vi "Partition_Sort.vi"(8 "FreezeIdx":i32[](array[numeric]), 9 "PartitionArray":string[](array[string]), 10 "FreezeTemps":dbl[](array[numeric]), 11 "Temps":dbl[][](array[numeric])) -> (0 "Freeze Idx / Part Array":i32[][](array[numeric]), 1 "Freeze / Part Array":bool[][](array[boolean]), 2 "FreezeTenos / Part Array":dbl[][](array[numeric]), 3 "MaxSize":i32)   [LabVIEW 2020]
uses:
  162fd0d4-48cb-478f-89f4-36ef44532280.vi
  <vilib>/Comparison/Less/Less Functor/Less Functor.lvclass
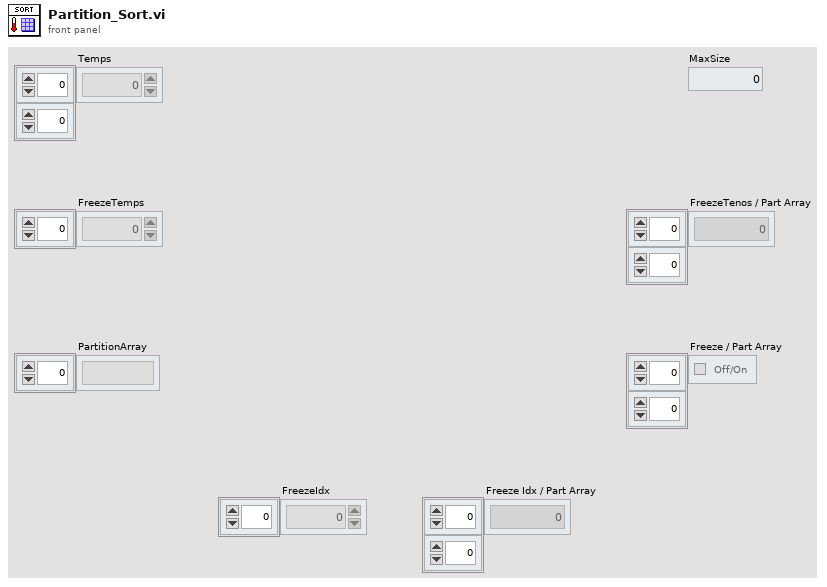
[diagram p1: front panel]
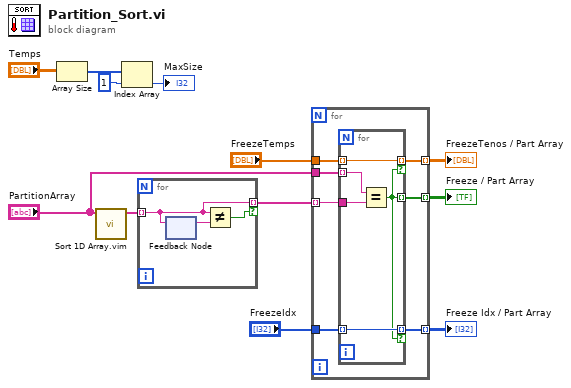
[diagram p0: block diagram]
diagram:
  n1 = Array Size(array="Temps") -> (size(s)=w9:i32[])
  n2 = call "Sort 1D Array.vim"("unsorted array"="PartitionArray") -> ("sorted array"=w2:string[])  [unwired: 10 in]
  n3 = Index Array(array=w9, index=1) -> (element=→"MaxSize":i32)
  n4 = for {
    tunnel: w2 -> [w13] mode=indexing
    tunnel: [w13] -> w3 mode=indexing if=w15
    n5 = feedback-in #1(w13) -> ()
    n6 = feedback #1() -> (w14:string)  [unwired: 1 in]
    n7 = Not Equal?(x=w13, y=w14) -> (x != y?=w15:bool)
  }
  n8 = for {
    tunnel: "PartitionArray" -> [w22]
    tunnel: "FreezeTemps" -> [w21]
    tunnel: w3 -> [w20] mode=indexing
    tunnel: [w19] -> w4 mode=indexing
    tunnel: [w18] -> w5 mode=indexing
    tunnel: "FreezeIdx" -> [w17]
    tunnel: [w16] -> w11 mode=indexing
    n9 = for {
      tunnel: w22 -> [w27] mode=indexing
      tunnel: w21 -> [w25] mode=indexing
      tunnel: w20 -> [w26]
      tunnel: [w25] -> w19 mode=indexing if=w23
      tunnel: [w23] -> w18 mode=indexing
      tunnel: w17 -> [w24] mode=indexing
      tunnel: [w24] -> w16 mode=indexing if=w23
      n10 = Equal?(x=w27, y=w26) -> (x = y?=w23:bool)
    }
  }
  "Freeze Idx / Part Array" <- w11
  "Freeze / Part Array" <- w5
  "FreezeTenos / Part Array" <- w4
